vi "initialize.vi"(4 "error in (no error)":errorcluster) -> (0 "error out":errorcluster, 1 "py interface file":path, 3 "Python session out":refnum<k35>)   [LabVIEW 2022 SP3]
panel:
  in  "relative py interface path":string="../bapsf_motion_interface.py"
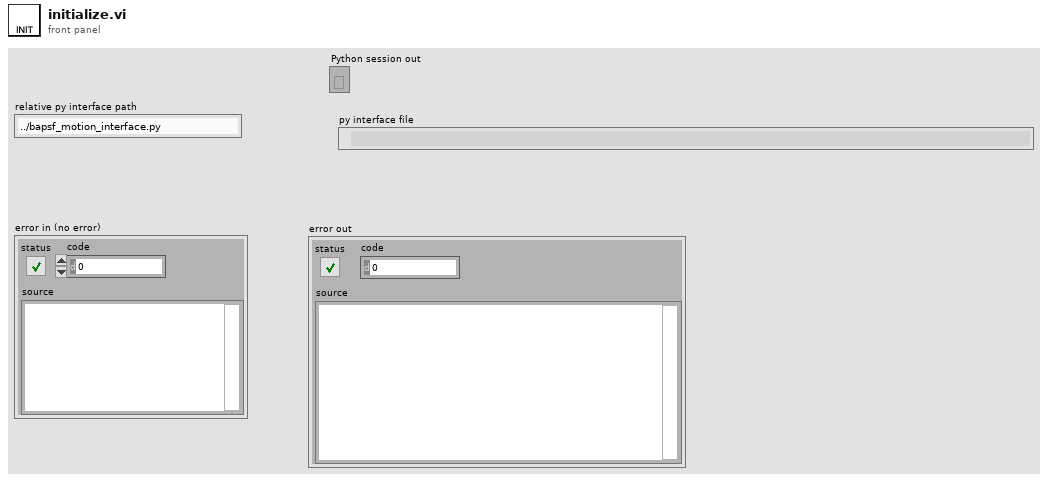
[diagram p1: front panel]
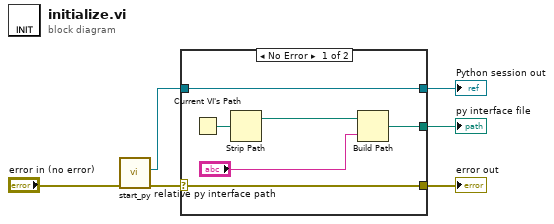
[diagram p0: block diagram]
diagram:
  n1 = call "start_py.vi"("error in"="error in (no error)") -> ("error out"=w1:errorcluster, "Python session"=w3:refnum<k35>)  [unwired: 5 in]
  n2 = case shown="No Error" w1 {
    selector: w1 -> [w8 w13]
    tunnel: [w8 w13] -> w6
    tunnel: [w9 _] -> w5
    tunnel: w3 -> [w7 w14]
    tunnel: [w7 w14] -> w2
    frame No Error {
      n3 = Current VI's Path() -> (path=w11:path)
      n4 = Strip Path(path=w11) -> (stripped path=w10:path)  [unwired: 1 out]
      n5 = Build Path(base path=w10, name or relative path="relative py interface path") -> (appended path=w9:path)
    }
    frame Error {
    }
  }
  "error out" <- w6
  "Python session out" <- w2
  "py interface file" <- w5
